vi "Main Page.vi"(8 "error in (no error)":errorcluster, 11 "Node Ptr":T3 format="%.0x") -> (0 "error out":errorcluster)   [LabVIEW 2019, in "Instrument Addon System Explorer.lvlib"]
uses:
  Instrument Addon System Explorer.lvlib
  <vilib>/NI VeriStand/Custom Device API/Custom Device Item Ref.ctl
  Shared/Types/FG Control.ctl
  <vilib>/NI/NI VeriStand Hardware Resource Discovery/_Types/Filter Type.ctl
  Shared/Constants.vi
  <vilib>/NI VeriStand/Custom Device API/NI VeriStand - Get Item Property.vi
  <vilib>/NI VeriStand/Custom Device API/Get Item Property (U32).vi
  <vilib>/NI VeriStand/Custom Device API/NI VeriStand - Set Item Property.vi
  <vilib>/NI VeriStand/Custom Device API/Set Item Property (U32).vi
  <vilib>/NI VeriStand/Custom Device API/Get Item Property (String).vi
  <vilib>/NI VeriStand/Custom Device API/Set Item Property (String).vi
  <vilib>/NI VeriStand/Custom Device API/Get Item Property (Boolean).vi
  <vilib>/NI VeriStand/Custom Device API/Set Item Property (Boolean).vi
  <vilib>/Utility/LVClass/Get LV Class Default Value.vi
  Protocols.lvlibp/Protocol Parent/Protocol Parent.lvclass
  <vilib>/NI VeriStand/Custom Device API/Custom Device API.lvlib
  Shared/Instrument Addon Shared.lvlib
  <vilib>/NI/NI VeriStand Hardware Resource Discovery/NIVS Hardware Discovery.lvlib
panel:
  out "Version":string
  in  "PCL Decimation":u32=1 min=1 max=10000 step=1
  in  "Protocol Settings":T1(tab)=enum."VISA"
  in  "COM Browse":bool
  in  "Termination Character":u8=10 format="%.0x"
  in  "End Write":bool=TRUE caption="End Write on Termination Character?"
  in  "End Read":bool=TRUE caption="End Read on Termination Character?"
  in  "XOFF":T2(ring)=enum."DC3"
  in  "XON":T2(ring)=enum."DC1"
  in  "Flow Control":u16(ring) items=["None"=0, "XON/XOFF"=1, "RTS/CTS"=2, "DTR/DSR"=4]
  in  "Stop Bits":u16(ring)=10 items=["1.0"=10, "1.5"=15, "2.0"=20]
  in  "Parity":enum16{"None", "Odd", "Even", "Mark", "Space"}(ring)
  in  "Data Bits":u16=8 min=5 max=8 step=1
  in  "Baud Rate":u32(ring)=9600 items=["75"=75, "110"=110, "134"=134, "150"=150, "300"=300, "600"=600, "1200"=1200, "1800"=1800, "2400"=2400, "4800"=4800, "7200"=7200, "9600"=9600, "14400"=14400, "19200"=19200, "28800"=28800, "38400"=38400, "56000"=56000, "57600"=57600, "115200"=115200, "128000"=128000, "230400"=230400, "460800"=460800, "921600"=921600, "1843200"=1843200, "3000000"=3000000]
  in  "Port":string="COM1"
  in  "VISA Browse":bool
  in  "Append Write Termination Character":bool caption="End Write on Termination Character?"
  in  "Timeout":u32=2000 caption="Timeout (ms)"
  in  "Termination Character":u8=10 format="%.0x"
  in  "Enable Termination Character":bool=TRUE caption="Enable Termination Character?"
  in  "VISA Resource":string="GPIB0::2::INSTR"
  in  "Port":u16
  in  "IP Address":string="localhost"
  in  "UDP Browse":bool
  in  "Target Port":u16
  in  "Target IP Address":string="localhost"
  in  "Local Port":u16
  in  "Local IP Address":string="localhost"
  in  "Assert Ren w/ IFC":bool=TRUE caption="Enable Termination Character?"
  in  "IST Bit Sense":bool=TRUE caption="Enable Termination Character?"
  in  "System Controller":bool=TRUE caption="Enable Termination Character?"
  in  "GPIB Address":string="1"
  in  "ConvBox Address":string="0"
  in  "ConvBox Browse":bool
  in  "Port":string="COM1"
  in  "Protocol":string(combo)
  in  "SHDocVw.IWebBrowser":refnum<k7>(container)
  in  "Header":cluster{"Section Name":string}={"Section Name"="Custom Device Item Settings"}
  in  "Description":string
  in  "Name":string
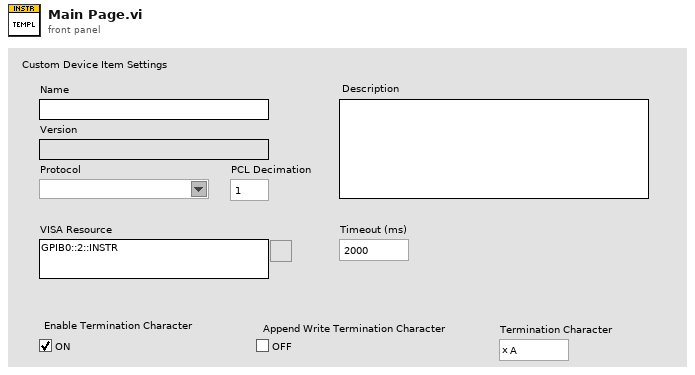
[diagram p1: front panel]
types:
  T1 = enum32{"RS232", "VISA", "TCP/IP", "UDP", "GPIB ConvBox"}
  T2 = enum16{"NUL", "SOH", "STX", "ETX", "EOT", "ENQ", "ACK", "BEL", "BS", "HT", "LF", "VT", "FF", "CR", "SO", "SI", "DLE", "DC1", "DC2", "DC3", "DC4", "NAK", "SYN", "ETB", "CAN", "EM", "SUB", "ESC", "FS", "GS", "RS", "US", "SP", "!", "\"", "#", "$", "%", "&", "'", "(", ")", "*", "+", ",", "- (-)", ".", "/", "0", "1", "2", "3", "4", "5", "6", "7", "8", "9", ":", ";", "<", "=", ">", "?", "@", "A", "B", "C", "D", "E", "F", "G", "H", "I", "J", "K", "L", "M", "N", "O", "P", "Q", "R", "S", "T", "U", "V", "W", "X", "Y", "Z", "[", "\\", "]", "^", "_", "`", "a", "b", "c", "d", "e", "f", "g", "h", "i", "j", "k", "l", "m", "n", "o", "p", "q", "r", "s", "t", "u", "v", "w", "x", "y", "z", "{", "|", "}", "~"}
  T3 = typedef "Custom Device API.lvlib/Custom Device Item Ref.ctl" = u64
  T4 = typedef "Instrument Addon Shared.lvlib/FG Control.ctl" = enum16{"Get", "Set"}
  T5 = typedef "Custom Device API.lvlib/Custom Device Item Info.ctl" = cluster{"Name":string, "Is Channel":bool, "GUID":string, "Is Waveform":bool}
  T6 = typedef "NIVS Hardware Discovery.lvlib/Filter Type.ctl" = enum16{"Device Category", "Product Name", "Ethernet", "XNET", "VISA", "FPGA", "EtherCAT Master", "DAQmx", "GPIB", "Serial"}
  T7 = typedef "Custom Device API.lvlib/Custom Device Commands.ctl" = enum16{"Default", "Item renamed", "Shutdown", "Dynamic button pressed"}
  T8 = typedef "Instrument Addon Shared.lvlib/VISA Settings.ctl" = cluster{"VISA Resource":string, "Enable Termination Character":bool, "Termination Character":u8, "Timeout":u32, "Append Write Termination Character":bool}
  T9 = typedef "Instrument Addon Shared.lvlib/TCPIP Settings.ctl" = cluster{"IP Address":string, "Port":u16}
  T10 = typedef "Instrument Addon Shared.lvlib/GPIB ConvBox Settings.ctl" = cluster{"Port":string, "ConvBox Address":string, "Assert Ren with IFC":bool, "System controller":bool, "IST bit sense":bool, "GPIB Address":string}
  T11 = typedef "Instrument Addon Shared.lvlib/UDP Settings.ctl" = cluster{"Local IP Address":string, "Local Port":u16, "Target IP Address":string, "Target Port":u16}
  T12 = typedef "Instrument Addon Shared.lvlib/RSXXX Port Settings.ctl" = cluster{"Port":string, "Baud Rate":u32, "Data Bits":u16, "Parity":enum16{"None", "Odd", "Even", "Mark", "Space"}, "Stop Bits":u16, "Flow Control":u16, "XON":enum16{"NUL", "SOH", "STX", "ETX", "EOT", "ENQ", "ACK", "BEL", "BS", "HT", "LF", "VT", "FF", "CR", "SO", "SI", "DLE", "DC1", "DC2", "DC3", "DC4", "NAK", "SYN", "ETB", "CAN", "EM", "SUB", "ESC", "FS", "GS", "RS", "US", "SP", "!", "\"", "#", "$", "%", "&", "'", "(", ")", "*", "+", ",", "- (-)", ".", "/", "0", "1", "2", "3", "4", "5", "6", "7", "8", "9", ":", ";", "<", "=", ">", "?", "@", "A", "B", "C", "D", "E", "F", "G", "H", "I", "J", "K", "L", "M", "N", "O", "P", "Q", "R", "S", "T", "U", "V", "W", "X", "Y", "Z", "[", "\\", "]", "^", "_", "`", "a", "b", "c", "d", "e", "f", "g", "h", "i", "j", "k", "l", "m", "n", "o", "p", "q", "r", "s", "t", "u", "v", "w", "x", "y", "z", "{", "|", "}", "~"}, "XOFF":enum16{"NUL", "SOH", "STX", "ETX", "EOT", "ENQ", "ACK", "BEL", "BS", "HT", "LF", "VT", "FF", "CR", "SO", "SI", "DLE", "DC1", "DC2", "DC3", "DC4", "NAK", "SYN", "ETB", "CAN", "EM", "SUB", "ESC", "FS", "GS", "RS", "US", "SP", "!", "\"", "#", "$", "%", "&", "'", "(", ")", "*", "+", ",", "- (-)", ".", "/", "0", "1", "2", "3", "4", "5", "6", "7", "8", "9", ":", ";", "<", "=", ">", "?", "@", "A", "B", "C", "D", "E", "F", "G", "H", "I", "J", "K", "L", "M", "N", "O", "P", "Q", "R", "S", "T", "U", "V", "W", "X", "Y", "Z", "[", "\\", "]", "^", "_", "`", "a", "b", "c", "d", "e", "f", "g", "h", "i", "j", "k", "l", "m", "n", "o", "p", "q", "r", "s", "t", "u", "v", "w", "x", "y", "z", "{", "|", "}", "~"}, "End Read on Termination Character":bool, "End Write on Termination Character":bool, "Termination Character":u8}
  T13 = typedef "Protocols.lvlibp/Protocol Parent.lvclass/Base Protocol Type.ctl" = enum16{"RS-XXX", "VISA", "TCPIP", "UDP", "GPIB ConvBox"}
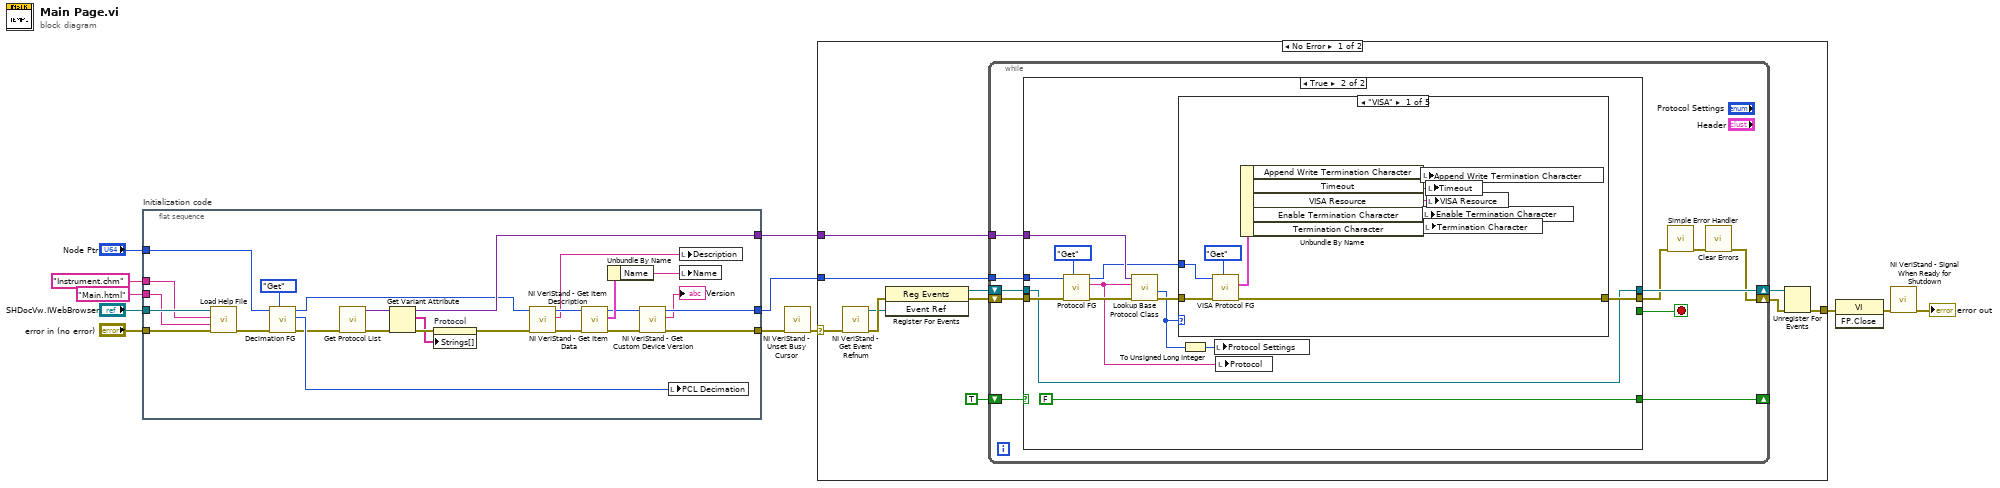
[diagram p0: block diagram]
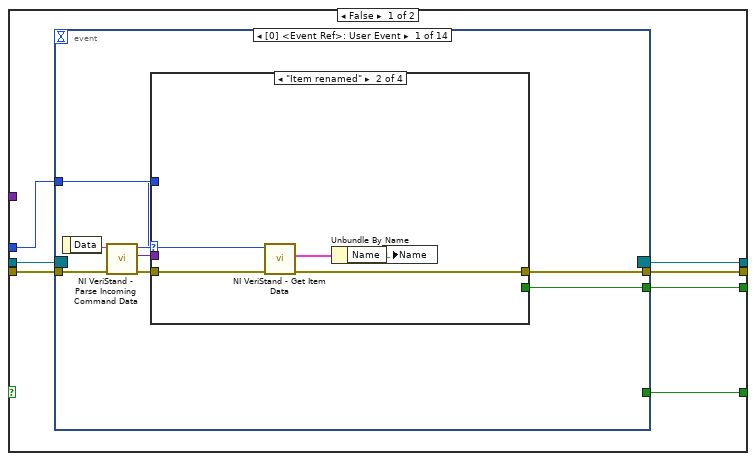
[diagram p2: hidden frame]
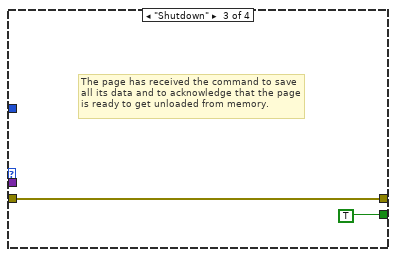
[diagram p4: hidden frame]
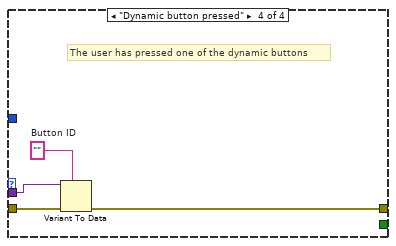
[diagram p5: hidden frame]
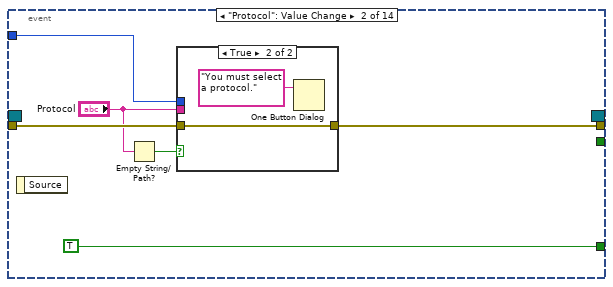
[diagram p6: hidden frame]
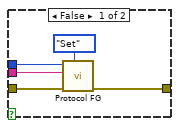
[diagram p7: hidden frame]
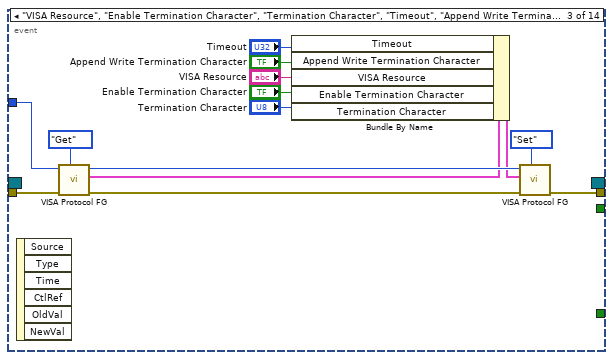
[diagram p8: hidden frame]
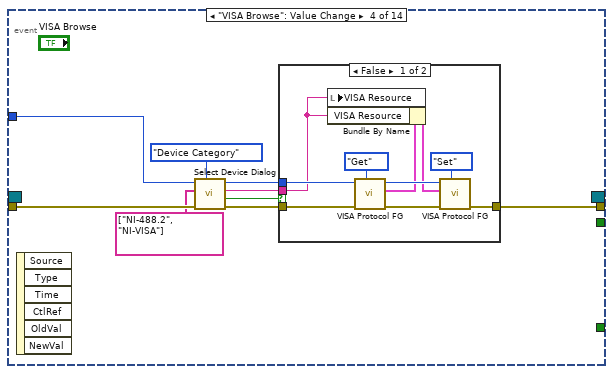
[diagram p9: hidden frame]
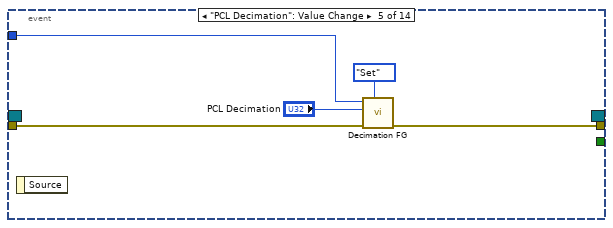
[diagram p11: hidden frame]
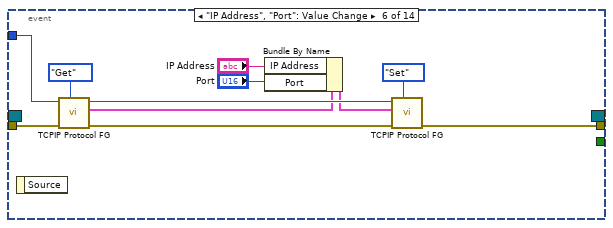
[diagram p12: hidden frame]
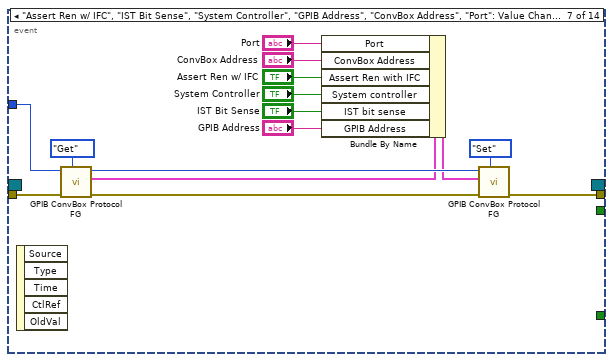
[diagram p13: hidden frame]
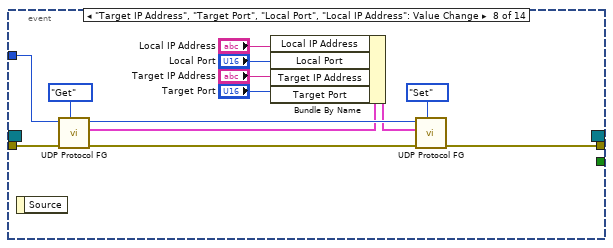
[diagram p14: hidden frame]
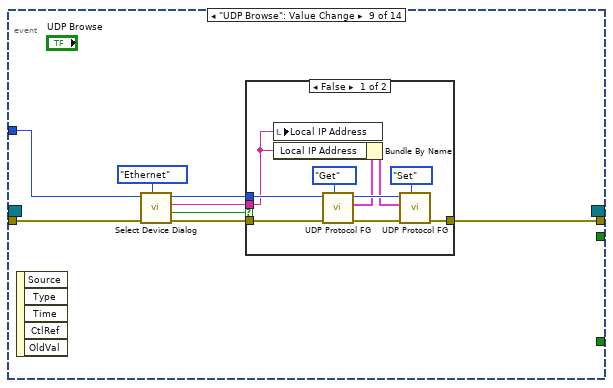
[diagram p15: hidden frame]
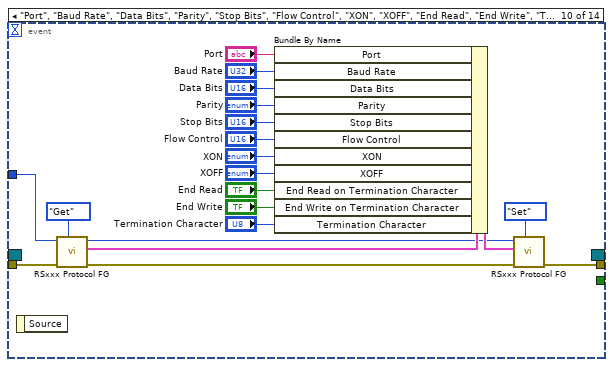
[diagram p17: hidden frame]
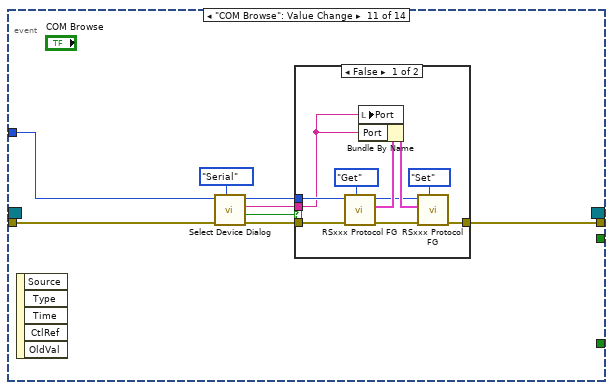
[diagram p18: hidden frame]
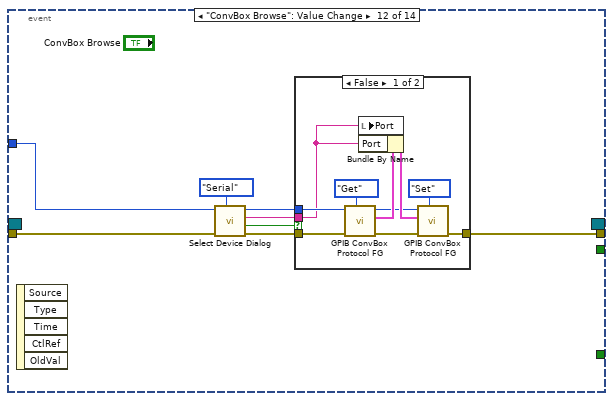
[diagram p20: hidden frame]
diagram:
  n1 = flat-sequence "Initialization code" {
    tunnel: "error in (no error)" -> [w33]
    tunnel: "Node Ptr" -> [w29]
    tunnel: [w16] -> w8
    tunnel: [w14] -> w5
    tunnel: "SHDocVw.IWebBrowser" -> [w32]
    tunnel: "Main.html" ("HTML File") -> [w31]
    tunnel: "Instrument.chm" ("Main CHM File") -> [w30]
    tunnel: [w21] -> w1
    frame #0 {
      n2 = call "Load Help File.vi"("error in (no error)"=w33, "HTML File"=w31, "Main CHM File"=w30, "SHDocVw.IWebBrowser2"=w32) -> ("error out"=w28:errorcluster)  [unwired: 7 in]
      n3 = call "Decimation FG.vi"("Action"=FG_Control."Get", "error in (no error)"=w28, "Device Item Ref in"=w29) -> ("error out"=w19:errorcluster, "Decimation out"=w26:u32, "Item Ref out"=w18:T3)  [unwired: 6 in]
      n4 = call "Get Protocol List.vi"("error in (no error)"=w19) -> ("error out"=w24:errorcluster, "Class Lookup"=w25:variant)  [unwired: 9 in]
      n5 = Get Variant Attribute(Variant=w25, error in=w24) -> (duplicate Variant=w21:variant, names=w22:string[], error out=w23:errorcluster)  [unwired: 2 in, 1 out]
      n6 = property on="Protocol" class="CmbBox"(error in=w23, "Strings[]"=w22) -> (error out=w20:errorcluster)  [unwired: 1 in, 1 out]
      n7 = call <vilib>:"NI VeriStand - Get Item Description.vi"("error in (no error)"=w20, "Item Ref in"=w18) -> ("error out"=w36:errorcluster, "Description"=w37:string, "Item Ref out"=w38:T3)  [unwired: 7 out]
      n8 = call <vilib>:"NI VeriStand - Get Item Data.vi"("error in (no error)"=w36, "Item Ref in"=w38) -> ("error out"=w17:errorcluster, "Item Info"=w35:T5, "Item Ref out"=w15:T3)  [unwired: 7 out]
      n9 = Unbundle By Name(w35) -> ("Name"=w34:string)
      n10 = call <vilib>:"NI VeriStand - Get Custom Device Version.vi"("error in (no error)"=w17, "Device Ref in"=w15) -> ("error out"=w16:errorcluster, "Value"=→"Version":string, "Device Ref out"=w14:T3)  [unwired: 7 in]
      n11 = local write "PCL Decimation"(w26) -> ()
      n12 = local write "Description"(w37) -> ()
      n13 = local write "Name"(w34) -> ()
    }
  }
  n14 = call <vilib>:"NI VeriStand - Unset Busy Cursor.vi"("error in (no error)"=w8) -> ("error out"=w7:errorcluster)  [unwired: 10 out]
  n15 = case shown="No Error" w7 {
    selector: w7 -> [w41 w332]
    tunnel: [w46 w330] -> w12
    tunnel: w5 -> [w42 _]
    tunnel: w1 -> [w40 _]
    frame No Error {
      n16 = call <vilib>:"NI VeriStand - Get Event Refnum.vi"("error in (no error)"=w41) -> ("error out"=w49:errorcluster, "Event Ref"=w45:refnum<user-event>)  [unwired: 9 out]
      n17 = register-events(error in=w49, w45) -> (reference out=w43:refnum<event-registration>, error out=w44:errorcluster)  [unwired: 1 in]
      n18 = while {
        tunnel: w42 -> [w56]
        shift-right: [w53] -> w47
        shift-left: w44 -> [w59]
        shift-right: [w60] -> w48
        shift-left: w43 -> [w58]
        tunnel: w40 -> [w52]
        shift-right: [w50] -> _
        shift-left: TRUE -> [w51]
        stop <- w57 stop-if-true
        n19 = case shown="True" w51 {
          tunnel: [w67 w266] -> w60
          tunnel: w59 -> [w66 w275]
          tunnel: w58 -> [w65 w266]
          tunnel: [w64 _] -> w57
          tunnel: w56 -> [w63 w274]
          tunnel: [w62 w267] -> w55
          tunnel: w52 -> [_ w272]
          tunnel: [w61 FALSE] -> w50
          frame False {
            n20 = event shown="[0] <Event Ref>: User Event" {
              selector: w65 -> [_ _ _ _ _ _ _ _ _ _ _ _ _ _]
              dyn-events: [_ _ _ _ _ _ _ _ _ _ _ _ _ _] -> w67
              timeout: _ -> [_ _ _ _ _ _ _ _ _ _ _ _ _ _]
              tunnel: w66 -> [w75 w92 w113 w122 w138 w149 w165 w177 w185 w214 w224 w243 w259 w262]
              tunnel: [w71 _ _ _ _ _ _ _ _ _ _ _ _ _] -> w64
              tunnel: [w70 w88 w109 w123 w136 w145 w162 w173 w186 w216 w225 w244 w258 w261] -> w62
              tunnel: w63 -> [w69 w93 w112 w120 w137 w148 w164 w176 w183 w212 w223 w242 w257 w263]
              tunnel: [_ TRUE _ _ _ _ _ _ _ _ _ _ _ _] -> w61
              event User Event {
                n21 = event-data() -> ("Data"=w74:string)  [unwired: 1 out]
                n22 = call <vilib>:"NI VeriStand - Parse Incoming Command Data.vi"("error in (no error)"=w75, "Incoming data"=w74) -> ("error out"=w73:errorcluster, "Outgoing data"=w68:variant, "Action"=w72:T7)  [unwired: 7 out]
                n23 = case shown="\"Item renamed\"" w72 {
                  tunnel: w73 -> [w76 w81 w82 w87]
                  tunnel: [_ _ TRUE _] -> w71
                  tunnel: [w76 w78 w82 w84] -> w70
                  tunnel: w69 -> [_ w80 _ _]
                  tunnel: w68 -> [_ _ _ w86]
                  frame "Default", Default {
                  }
                  frame "Item renamed" {
                    n24 = call <vilib>:"NI VeriStand - Get Item Data.vi"("error in (no error)"=w81, "Item Ref in"=w80) -> ("error out"=w78:errorcluster, "Item Info"=w79:T5)  [unwired: 8 out]
                    n25 = Unbundle By Name(w79) -> ("Name"=w77:string)
                    n26 = local write "Name"(w77) -> ()
                  }
                  frame "Shutdown" {
                    # "The page has received the command to save all its data and to acknowledge that the page is ready to get unloaded from memory."
                  }
                  frame "Dynamic button pressed" {
                    w85 = ""  # Button ID
                    # "The user has pressed one of the dynamic buttons"
                    n27 = Variant To Data(error in=w87, type=w85, Variant=w86) -> (error out=w84:errorcluster)  [unwired: 1 out]
                  }
                }
              }
              event "Protocol": Value Change {
                n28 = event-data() -> ()  [unwired: 2 out]
                n29 = Empty String/Path?(string/path="Protocol") -> (empty?=w90:bool)
                n30 = case shown="True" w90 {
                  tunnel: w93 -> [w96 _]
                  tunnel: w92 -> [w97 w99]
                  tunnel: [w94 w99] -> w88
                  tunnel: "Protocol" -> [w95 _]
                  frame False {
                    n31 = call "Protocol FG.vi"("Action"=FG_Control."Set", "error in (no error)"=w97, "Protocol"=w95, "Device Item Ref in"=w96) -> ("error out"=w94:errorcluster)  [unwired: 5 in, 2 out]
                  }
                  frame True {
                    n32 = One Button Dialog(message="You must select a protocol.") -> ()  [unwired: 1 in, 1 out]
                  }
                }
              }
              event "VISA Resource", "Enable Termination Character", "Termination Character", "Timeout", "Append Write Termination Character": Value Change {
                n33 = event-data() -> ()  [unwired: 7 out]
                n34 = call "VISA Protocol FG.vi"("Action"=FG_Control."Get", "error in (no error)"=w113, "Device Item Ref in"=w112) -> ("error out"=w110:errorcluster, "VISA Config"=w107:T8, "Item Ref out"=w108:T3)  [unwired: 6 in]
                n35 = Bundle By Name(cluster=w107, "Timeout"="Timeout", "Append Write Termination Character"="Append Write Termination Character", "VISA Resource"="VISA Resource", "Enable Termination Character"="Enable Termination Character", "Termination Character"="Termination Character") -> (w106:T8)
                n36 = call "VISA Protocol FG.vi"("Action"=FG_Control."Set", "error in (no error)"=w110, "VISA Config"=w106, "Device Item Ref in"=w108) -> ("error out"=w109:errorcluster)  [unwired: 5 in, 2 out]
              }
              event "VISA Browse": Value Change {
                n37 = event-data() -> ()  [unwired: 7 out]
                n38 = call <vilib>:"Select Device Dialog.vi"("Filter Type"=Filter_Type."Device Category", "error in (no error)"=w122, "Filter Names"=string[] ["NI-488.2", "NI-VISA"], "Item Ref in"=w120) -> ("error out"=w121:errorcluster, "Cancelled?"=w118:bool, "Selected Alias"=w117:string, "Item Ref out"=w119:T3)  [unwired: 4 in]
                n39 = case shown="False" w118 {
                  tunnel: w121 -> [w132 w134]
                  tunnel: w119 -> [w131 _]
                  tunnel: [w128 w134] -> w123
                  tunnel: w117 -> [w124 _]
                  frame False {
                    n40 = local write "VISA Resource"(w124) -> ()
                    n41 = call "VISA Protocol FG.vi"("Action"=FG_Control."Get", "error in (no error)"=w132, "Device Item Ref in"=w131) -> ("error out"=w129:errorcluster, "VISA Config"=w126:T8, "Item Ref out"=w127:T3)  [unwired: 6 in]
                    n42 = Bundle By Name(cluster=w126, "VISA Resource"=w124) -> (w125:T8)
                    n43 = call "VISA Protocol FG.vi"("Action"=FG_Control."Set", "error in (no error)"=w129, "VISA Config"=w125, "Device Item Ref in"=w127) -> ("error out"=w128:errorcluster)  [unwired: 5 in, 2 out]
                  }
                  frame True {
                  }
                }
              }
              event "PCL Decimation": Value Change {
                n44 = event-data() -> ()  [unwired: 2 out]
                n45 = call "Decimation FG.vi"("Action"=FG_Control."Set", "error in (no error)"=w138, "Decimation"="PCL Decimation", "Device Item Ref in"=w137) -> ("error out"=w136:errorcluster)  [unwired: 5 in, 2 out]
              }
              event "IP Address", "Port": Value Change {
                n46 = event-data() -> ()  [unwired: 2 out]
                n47 = call "TCPIP Protocol FG.vi"("Action"=FG_Control."Get", "error in (no error)"=w149, "Device Item Ref in"=w148) -> ("error out"=w146:errorcluster, "TCP/IP Config"=w143:T9, "Item Ref out"=w144:T3)  [unwired: 6 in]
                n48 = Bundle By Name(cluster=w143, "IP Address"="IP Address", "Port"="Port") -> (w142:T9)
                n49 = call "TCPIP Protocol FG.vi"("Action"=FG_Control."Set", "error in (no error)"=w146, "TCP/IP Config"=w142, "Device Item Ref in"=w144) -> ("error out"=w145:errorcluster)  [unwired: 5 in, 2 out]
              }
              event "Assert Ren w/ IFC", "IST Bit Sense", "System Controller", "GPIB Address", "ConvBox Address", "Port": Value Change {
                n50 = event-data() -> ()  [unwired: 6 out]
                n51 = call "GPIB ConvBox Protocol FG.vi"("Action"=FG_Control."Get", "error in (no error)"=w165, "Device Item Ref in"=w164) -> ("error out"=w163:errorcluster, "GPIB ConvBox Config"=w159:T10, "Item Ref out"=w161:T3)  [unwired: 6 in]
                n52 = Bundle By Name(cluster=w159, "Port"="Port", "ConvBox Address"="ConvBox Address", "Assert Ren with IFC"="Assert Ren w/ IFC", "System controller"="System Controller", "IST bit sense"="IST Bit Sense", "GPIB Address"="GPIB Address") -> (w158:T10)
                n53 = call "GPIB ConvBox Protocol FG.vi"("Action"=FG_Control."Set", "error in (no error)"=w163, "GPIB ConvBox Config"=w158, "Device Item Ref in"=w161) -> ("error out"=w162:errorcluster)  [unwired: 5 in, 2 out]
              }
              event "Target IP Address", "Target Port", "Local Port", "Local IP Address": Value Change {
                n54 = event-data() -> ()  [unwired: 2 out]
                n55 = call "UDP Protocol FG.vi"("Action"=FG_Control."Get", "error in (no error)"=w177, "Device Item Ref in"=w176) -> ("error out"=w174:errorcluster, "UDP Config"=w171:T11, "Item Ref out"=w172:T3)  [unwired: 6 in]
                n56 = Bundle By Name(cluster=w171, "Local IP Address"="Local IP Address", "Local Port"="Local Port", "Target IP Address"="Target IP Address", "Target Port"="Target Port") -> (w170:T11)
                n57 = call "UDP Protocol FG.vi"("Action"=FG_Control."Set", "error in (no error)"=w174, "UDP Config"=w170, "Device Item Ref in"=w172) -> ("error out"=w173:errorcluster)  [unwired: 5 in, 2 out]
              }
              event "UDP Browse": Value Change {
                n58 = event-data() -> ()  [unwired: 6 out]
                n59 = call <vilib>:"Select Device Dialog.vi"("Filter Type"=Filter_Type."Ethernet", "error in (no error)"=w185, "Item Ref in"=w183) -> ("error out"=w184:errorcluster, "Cancelled?"=w181:bool, "Selected Alias"=w180:string, "Item Ref out"=w182:T3)  [unwired: 5 in]
                n60 = case shown="False" w181 {
                  tunnel: w184 -> [w195 w197]
                  tunnel: w182 -> [w194 _]
                  tunnel: [w191 w197] -> w186
                  tunnel: w180 -> [w187 _]
                  frame False {
                    n61 = local write "Local IP Address"(w187) -> ()
                    n62 = call "UDP Protocol FG.vi"("Action"=FG_Control."Get", "error in (no error)"=w195, "Device Item Ref in"=w194) -> ("error out"=w192:errorcluster, "UDP Config"=w189:T11, "Item Ref out"=w190:T3)  [unwired: 6 in]
                    n63 = Bundle By Name(cluster=w189, "Local IP Address"=w187) -> (w188:T11)
                    n64 = call "UDP Protocol FG.vi"("Action"=FG_Control."Set", "error in (no error)"=w192, "UDP Config"=w188, "Device Item Ref in"=w190) -> ("error out"=w191:errorcluster)  [unwired: 5 in, 2 out]
                  }
                  frame True {
                  }
                }
              }
              event "Port", "Baud Rate", "Data Bits", "Parity", "Stop Bits", "Flow Control", "XON", "XOFF", "End Read", "End Write", "Termination Character": Value Change {
                n65 = event-data() -> ()  [unwired: 2 out]
                n66 = call "RSxxx Protocol FG.vi"("Action"=FG_Control."Get", "error in (no error)"=w214, "Device Item Ref in"=w212) -> ("error out"=w213:errorcluster, "Serial Config"=w211:T12, "Item Ref out"=w198:T3)  [unwired: 6 in]
                n67 = Bundle By Name(cluster=w211, "Port"="Port", "Baud Rate"="Baud Rate", "Data Bits"="Data Bits", "Parity"="Parity", "Stop Bits"="Stop Bits", "Flow Control"="Flow Control", "XON"="XON", "XOFF"="XOFF", "End Read on Termination Character"="End Read", "End Write on Termination Character"="End Write", "Termination Character"="Termination Character") -> (w210:T12)
                n68 = call "RSxxx Protocol FG.vi"("Action"=FG_Control."Set", "error in (no error)"=w213, "Serial Config"=w210, "Device Item Ref in"=w198) -> ("error out"=w216:errorcluster)  [unwired: 5 in, 2 out]
              }
              event "COM Browse": Value Change {
                n69 = event-data() -> ()  [unwired: 6 out]
                n70 = call <vilib>:"Select Device Dialog.vi"("Filter Type"=Filter_Type."Serial", "error in (no error)"=w224, "Item Ref in"=w223) -> ("error out"=w221:errorcluster, "Cancelled?"=w220:bool, "Selected Alias"=w219:string, "Item Ref out"=w222:T3)  [unwired: 5 in]
                n71 = case shown="False" w220 {
                  tunnel: [w234 w236] -> w225
                  tunnel: w221 -> [w232 w236]
                  tunnel: w222 -> [w230 _]
                  tunnel: w219 -> [w226 _]
                  frame False {
                    n72 = call "RSxxx Protocol FG.vi"("Action"=FG_Control."Get", "error in (no error)"=w232, "Device Item Ref in"=w230) -> ("error out"=w231:errorcluster, "Serial Config"=w229:T12, "Item Ref out"=w227:T3)  [unwired: 6 in]
                    n73 = local write "Port"(w226) -> ()
                    n74 = Bundle By Name(cluster=w229, "Port"=w226) -> (w228:T12)
                    n75 = call "RSxxx Protocol FG.vi"("Action"=FG_Control."Set", "error in (no error)"=w231, "Serial Config"=w228, "Device Item Ref in"=w227) -> ("error out"=w234:errorcluster)  [unwired: 5 in, 2 out]
                  }
                  frame True {
                  }
                }
              }
              event "ConvBox Browse": Value Change {
                n76 = event-data() -> ()  [unwired: 6 out]
                n77 = call <vilib>:"Select Device Dialog.vi"("Filter Type"=Filter_Type."Serial", "error in (no error)"=w243, "Item Ref in"=w242) -> ("error out"=w240:errorcluster, "Cancelled?"=w239:bool, "Selected Alias"=w238:string, "Item Ref out"=w241:T3)  [unwired: 5 in]
                n78 = case shown="False" w239 {
                  tunnel: [w253 w255] -> w244
                  tunnel: w240 -> [w251 w255]
                  tunnel: w241 -> [w249 _]
                  tunnel: w238 -> [w245 _]
                  frame False {
                    n79 = call "GPIB ConvBox Protocol FG.vi"("Action"=FG_Control."Get", "error in (no error)"=w251, "Device Item Ref in"=w249) -> ("error out"=w250:errorcluster, "GPIB ConvBox Config"=w248:T10, "Item Ref out"=w246:T3)  [unwired: 6 in]
                    n80 = local write "Port"(w245) -> ()
                    n81 = Bundle By Name(cluster=w248, "Port"=w245) -> (w247:T10)
                    n82 = call "GPIB ConvBox Protocol FG.vi"("Action"=FG_Control."Set", "error in (no error)"=w250, "GPIB ConvBox Config"=w247, "Device Item Ref in"=w246) -> ("error out"=w253:errorcluster)  [unwired: 5 in, 2 out]
                  }
                  frame True {
                  }
                }
              }
              event "Name": Value Change {
                n83 = event-data() -> ()  [unwired: 2 out]
                n84 = call <vilib>:"NI VeriStand - Rename Custom Device Item.vi"("error in (no error)"=w259, "New Name"="Name", "Item Ref in"=w257) -> ("error out"=w258:errorcluster)  [unwired: 1 in, 7 out]
              }
              event "Description": Value Change {
                n85 = event-data() -> ()  [unwired: 2 out]
                n86 = call <vilib>:"NI VeriStand - Set Item Description.vi"("error in (no error)"=w262, "Description"="Description", "Item Ref in"=w263) -> ("error out"=w261:errorcluster)  [unwired: 8 out]
              }
            }
          }
          frame True {
            n87 = call "Protocol FG.vi"("Action"=FG_Control."Get", "error in (no error)"=w275, "Device Item Ref in"=w274) -> ("error out"=w271:errorcluster, "Protocol out"=w268:string, "Item Ref out"=w270:T3)  [unwired: 6 in]
            n88 = call "Lookup Base Protocol Class.vi"("error in (no error)"=w271, "Protocol in"=w268, "Class Lookup"=w272) -> ("error out"=w273:errorcluster, "Protocol out"=w265:T13)  [unwired: 5 in, 2 out]
            n89 = case shown="\"VISA\"" w265 {
              tunnel: w273 -> [w286 w293 w302 w318 w329]
              tunnel: [w285 w292 w301 w317 w328] -> w267
              tunnel: w270 -> [w284 w291 w300 w316 w327]
              frame "VISA" {
                n90 = call "VISA Protocol FG.vi"("Action"=FG_Control."Get", "error in (no error)"=w286, "Device Item Ref in"=w284) -> ("error out"=w285:errorcluster, "VISA Config"=w282:T8)  [unwired: 6 in, 1 out]
                n91 = Unbundle By Name(w282) -> ("Append Write Termination Character"=w277:bool, "Timeout"=w278:u32, "VISA Resource"=w281:string, "Enable Termination Character"=w280:bool, "Termination Character"=w279:u8)
                n92 = local write "Append Write Termination Character"(w277) -> ()
                n93 = local write "Enable Termination Character"(w280) -> ()
                n94 = local write "Termination Character"(w279) -> ()
                n95 = local write "Timeout"(w278) -> ()
                n96 = local write "VISA Resource"(w281) -> ()
              }
              frame "TCPIP" {
                n97 = call "TCPIP Protocol FG.vi"("Action"=FG_Control."Get", "error in (no error)"=w293, "Device Item Ref in"=w291) -> ("error out"=w292:errorcluster, "TCP/IP Config"=w289:T9)  [unwired: 6 in, 1 out]
                n98 = Unbundle By Name(w289) -> ("IP Address"=w288:string, "Port"=w287:u16)
                n99 = local write "IP Address"(w288) -> ()
                n100 = local write "Port"(w287) -> ()
              }
              frame "UDP" {
                n101 = call "UDP Protocol FG.vi"("Action"=FG_Control."Get", "error in (no error)"=w302, "Device Item Ref in"=w300) -> ("error out"=w301:errorcluster, "UDP Config"=w298:T11)  [unwired: 6 in, 1 out]
                n102 = Unbundle By Name(w298) -> ("Local IP Address"=w297:string, "Local Port"=w296:u16, "Target IP Address"=w295:string, "Target Port"=w294:u16)
                n103 = local write "Local IP Address"(w297) -> ()
                n104 = local write "Local Port"(w296) -> ()
                n105 = local write "Target IP Address"(w295) -> ()
                n106 = local write "Target Port"(w294) -> ()
              }
              frame "RS-XXX" {
                n107 = call "RSxxx Protocol FG.vi"("Action"=FG_Control."Get", "error in (no error)"=w318, "Device Item Ref in"=w316) -> ("error out"=w317:errorcluster, "Serial Config"=w314:T12)  [unwired: 6 in, 1 out]
                n108 = Unbundle By Name(w314) -> ("Port"=w313:string, "Baud Rate"=w312:u32, "Data Bits"=w303:u16, "Parity"=w304:enum16{"None", "Odd", "Even", "Mark", "Space"}, "Stop Bits"=w305:u16, "Flow Control"=w306:u16, "XON"=w307:T2, "XOFF"=w308:T2, "End Read on Termination Character"=w309:bool, "End Write on Termination Character"=w310:bool, "Termination Character"=w311:u8)
                n109 = local write "Termination Character"(w311) -> ()
                n110 = local write "Flow Control"(w306) -> ()
                n111 = local write "Data Bits"(w303) -> ()
                n112 = local write "Stop Bits"(w305) -> ()
                n113 = local write "XON"(w307) -> ()
                n114 = local write "End Write"(w310) -> ()
                n115 = local write "Port"(w313) -> ()
                n116 = local write "Baud Rate"(w312) -> ()
                n117 = local write "Parity"(w304) -> ()
                n118 = local write "XOFF"(w308) -> ()
                n119 = local write "End Read"(w309) -> ()
              }
              frame "GPIB ConvBox" {
                n120 = call "GPIB ConvBox Protocol FG.vi"("Action"=FG_Control."Get", "error in (no error)"=w329, "Device Item Ref in"=w327) -> ("error out"=w328:errorcluster, "GPIB ConvBox Config"=w325:T10)  [unwired: 6 in, 1 out]
                n121 = Unbundle By Name(w325) -> ("Port"=w324:string, "ConvBox Address"=w319:string, "Assert Ren with IFC"=w320:bool, "System controller"=w321:bool, "IST bit sense"=w322:bool, "GPIB Address"=w323:string)
                n122 = local write "Port"(w324) -> ()
                n123 = local write "ConvBox Address"(w319) -> ()
                n124 = local write "Assert Ren w/ IFC"(w320) -> ()
                n125 = local write "System Controller"(w321) -> ()
                n126 = local write "IST Bit Sense"(w322) -> ()
                n127 = local write "GPIB Address"(w323) -> ()
              }
            }
            n128 = To Unsigned Long Integer(number=w265) -> (unsigned 32bit integer=w269:u32)
            n129 = local write "Protocol Settings"(w269) -> ()
            n130 = local write "Protocol"(w268) -> ()
          }
        }
        n131 = call <vilib>:"Simple Error Handler.vi"("error in (no error)"=w55) -> ("error out"=w54:errorcluster)  [unwired: 1 in, 7 out]
        n132 = call <vilib>:"Clear Errors.vi"("error in (no error)"=w54) -> ("error out"=w53:errorcluster)  [unwired: 1 in, 5 out]
      }
      n133 = Unregister For Events(event registration refnum=w48, error in=w47) -> (error out=w46:errorcluster)
    }
    frame Error {
      n134 = call <vilib>:"Simple Error Handler.vi"("error in (no error)"=w332) -> ("error out"=w331:errorcluster)  [unwired: 1 in, 7 out]
      n135 = call <vilib>:"Clear Errors.vi"("error in (no error)"=w331) -> ("error out"=w330:errorcluster)  [unwired: 1 in, 5 out]
    }
  }
  n136 = invoke class="VI" method="FP.Close"(error in=w12) -> (error out=w11:errorcluster)  [unwired: 2 in, 2 out]
  n137 = call <vilib>:"NI VeriStand - Signal When Ready for Shutdown.vi"("error in (no error)"=w11) -> ("error out"=→"error out":errorcluster)  [unwired: 10 out]
